vi "VIReference.vi"(1 "Fact In":refnum<class "Fact.lvclass">) -> (0 "VI Refnum":refnum<vi>)   [LabVIEW 2019, in "TestCase.lvlib" / "Fact.lvclass"]
uses:
  Fact.lvclass
  Fact.lvclass/Fact.ctl
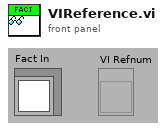
[diagram p1: front panel]
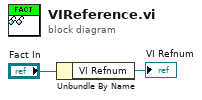
[diagram p0: block diagram]
diagram:
  n1 = Unbundle By Name("Fact In") -> ("VI Refnum"=→"VI Refnum":refnum<vi>)
